vi "UnscentedKalmanFilter_New.vi"(5 "States":i32, 6 "dt_Seconds":dbl=0.02, 7 "Outputs":i32, 8 "UNSCENTED_KALMAN_NEW_FUNC_GROUP":T1, 10 "MeasurementStdDevs":T3, 11 "StateStdDevs":T3) -> (0 "Error":bool, 3 "UnscentedKalmanFiilter":T4)   [LabVIEW 2019, in "Trajectory_Library.lvlib"]
doc: "Creates a new LINEAR SYSTEM data cluster with the specified values. \n\n\nInputs: \n - XXX -- XXX.\n\nOutputs:\n - XXX -- XXX."
uses:
  Trajectory_Library.lvlib
  UNSCENTED_KALMAN_FILTER.ctl
  <vilib>/Analysis/Matrix/Datatypes/RealMatrix.ctl
  MERWE_SCALED_SIGMA_PTS.ctl
  BiFunction_FUNC_TYPE.ctl
  UNSCENTED_KALMAN_NEW_FUNC_GROUP.ctl
  MatrixHelper_CoerceSize.vi
  <vilib>/Analysis/Matrix/NI_Matrix.lvlib
panel:
  # "<States,1>"
  # "<Outputs,1>"
  # "State Estimate <Statess,1>"
  # "<States, States>"
  # "<States, ?>"
  # "<Statess,  States>"
  # "<Outputs, Outputs>"
  # "<?, 1>"
  # "<?, 1>"
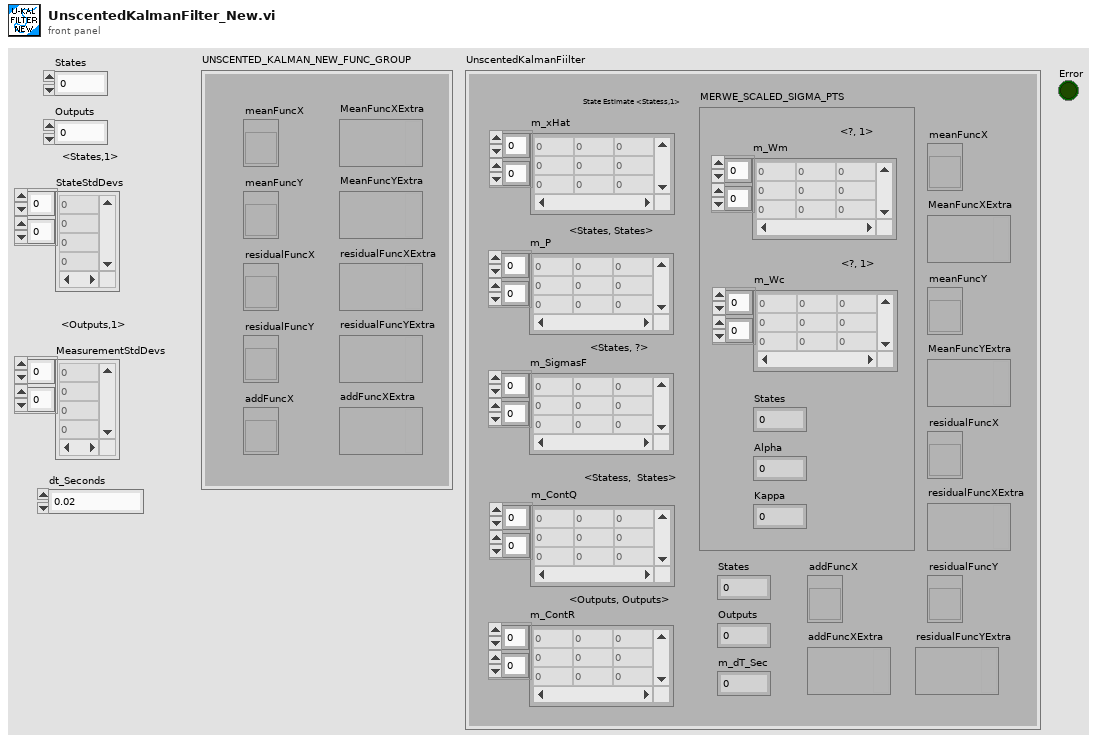
[diagram p1: front panel]
types:
  T1 = typedef "Trajectory_Library.lvlib/UNSCENTED_KALMAN_NEW_FUNC_GROUP.ctl" = cluster{"meanFuncX":T2, "meanFuncY":T2, "residualFuncX":T2, "residualFuncY":T2, "addFuncX":T2, "MeanFuncXExtra":variant, "MeanFuncYExtra":variant, "residualFuncXExtra":variant, "residualFuncYExtra":variant, "addFuncXExtra":variant}
  T2 = typedef "Trajectory_Library.lvlib/BiFunction_FUNC_TYPE.ctl" = refnum<vi>
  T3 = typedef "NI_Matrix.lvlib/RealMatrix.ctl" = dbl[][]
  T4 = typedef "Trajectory_Library.lvlib/UNSCENTED_KALMAN_FILTER.ctl" = cluster{"m_P":T3, "m_xHat":T3, "States":i32, "Outputs":i32, "m_ContR":T3, "m_ContQ":T3, "m_SigmasF":T3, "m_dT_Sec":dbl, "MERWE_SCALED_SIGMA_PTS":T5, "meanFuncX":T2, "meanFuncY":T2, "residualFuncX":T2, "residualFuncY":T2, "addFuncX":T2, "addFuncXExtra":variant, "residualFuncYExtra":variant, "residualFuncXExtra":variant, "MeanFuncYExtra":variant, "MeanFuncXExtra":variant}
  T5 = typedef "Trajectory_Library.lvlib/MERWE_SCALED_SIGMA_PTS.ctl" = cluster{"m_Wm":T3, "States":i32, "Alpha":dbl, "m_Wc":T3, "Kappa":i32}
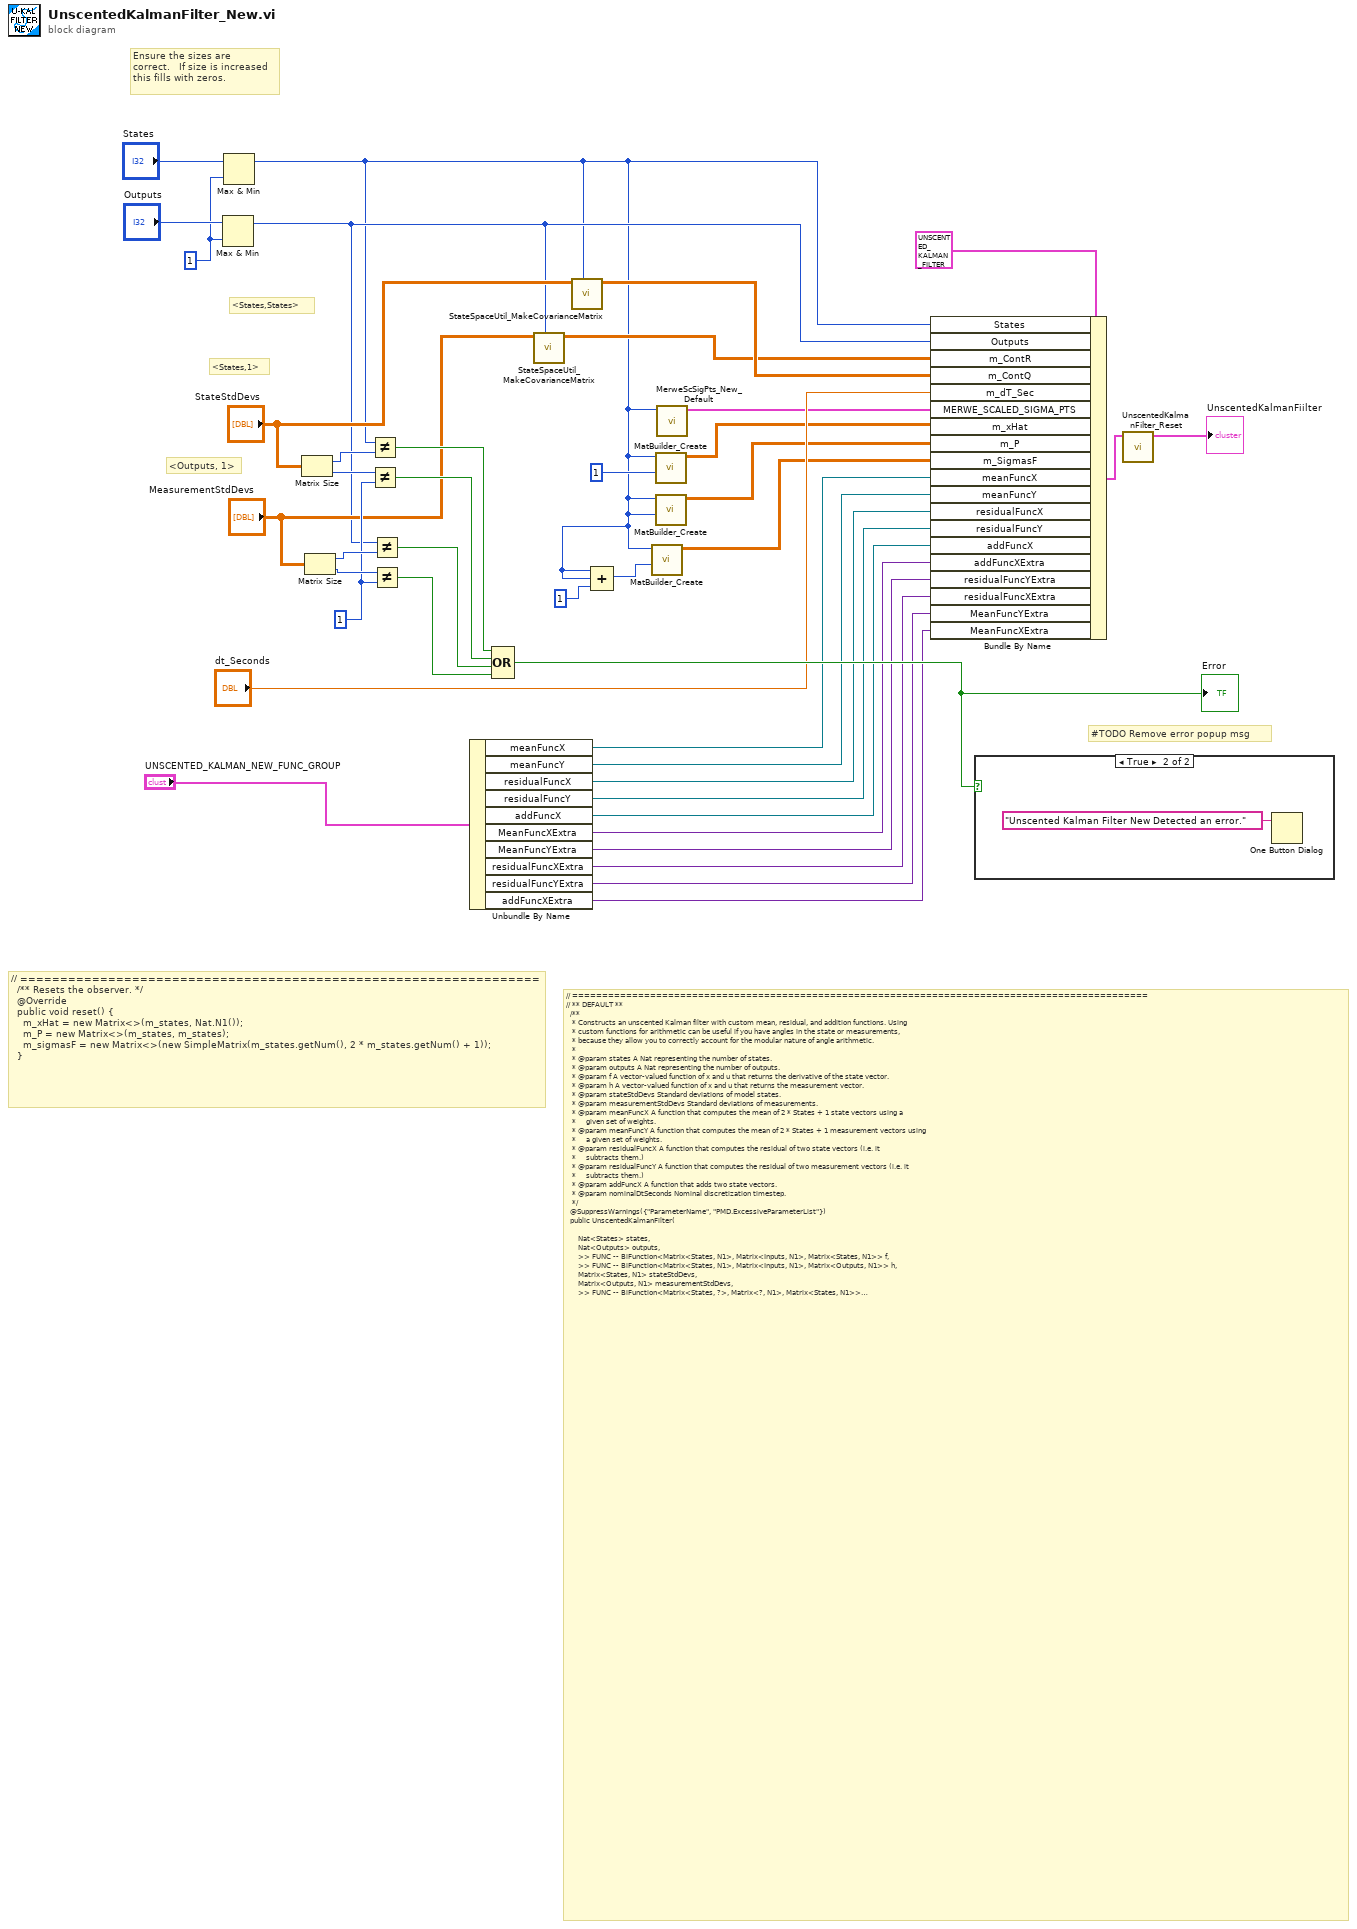
[diagram p0: block diagram]
diagram:
  w30 = 1 ("y")
  w39 = 1 ("y")
  # "// =================================================================\n  /** Resets the observer. */\n  @Override\n  public void reset() {\n    m_xHat = new Matrix<>(m_states, Nat.N1());\n    m_P = new Matrix<>(m_states, m_states);\n    m_sigmasF = new Matrix<>(new SimpleMatrix(m_states.getNum(), 2 * m_states.getNum() + 1));\n  }"
  # "// ================================================================================================\n// ** DEFAULT **\n  /**\n   * Constructs an unscented Kalman filter with custom mean, residual, and addition functions. Using\n   * custom functions for arithmetic can be useful if you have angles in the state or measurements,\n   * because they allow you to correctly account for the modular nature of angle arithmetic.\n   *\n   * @param states A Nat representing the number of states.\n   * @param outputs A Nat representing the number of outputs.\n   * @param f A vector-valued function of x and u that returns the derivative of the state vector.\n   * @param h A vector-valued function of x and u that returns the measurement vector.\n   * @param stateStdDevs Standard deviations of model states.\n   * @param measurementStdDevs Standard deviations of measurements.\n   * @param meanFuncX A function that computes the mean of 2 * States + 1 state vectors using a\n   *     given set of weights.\n   * @param meanFuncY A function that computes the mean of 2 * States + 1 measurement vectors using\n   *     a given set of weights.\n   * @param residualFuncX A function that computes the residual of two state vectors (i.e. it\n   *     subtracts them.)\n   * @param residualFuncY A function that computes the residual of two measurement vectors (i.e. it\n   *     subtracts them.)\n   * @param addFuncX A function that adds two state vectors.\n   * @param nominalDtSeconds Nominal discretization timestep.\n   */\n  @SuppressWarnings({\"ParameterName\", \"PMD.ExcessiveParameterList\"})\n  public UnscentedKalmanFilter(\n\n      Nat<States> states,\n      Nat<Outputs> outputs,\n      >> FUNC -- BiFunction<Matrix<States, N1>, Matrix<Inputs, N1>, Matrix<States, N1>> f,\n      >> FUNC -- BiFunction<Matrix<States, N1>, Matrix<Inputs, N1>, Matrix<Outputs, N1>> h,\n      Matrix<States, N1> stateStdDevs,\n      Matrix<Outputs, N1> measurementStdDevs,\n      >> FUNC -- BiFunction<Matrix<States, ?>, Matrix<?, N1>, Matrix<States, N1>> meanFuncX,\n      >> FUNC -- BiFunction<Matrix<Outputs, ?>, Matrix<?, N1>, Matrix<Outputs, N1>> meanFuncY,\n      >> FUNC -- BiFunction<Matrix<States, N1>, Matrix<States, N1>, Matrix<States, N1>> residualFuncX,\n      >> FUNC -- BiFunction<Matrix<Outputs, N1>, Matrix<Outputs, N1>, Matrix<Outputs, N1>> residualFuncY,\n      >> FUNC -- BiFunction<Matrix<States, N1>, Matrix<States, N1>, Matrix<States, N1>> addFuncX,\n      double nominalDtSeconds) {\n\n    this.m_states = states;\n    this.m_outputs = outputs;\n\n    m_f = f;\n    m_h = h;\n\n    m_meanFuncX = meanFuncX;\n    m_meanFuncY = meanFuncY;\n    m_residualFuncX = residualFuncX;\n    m_residualFuncY = residualFuncY;\n    m_addFuncX = addFuncX;\n\n    m_dtSeconds = nominalDtSeconds;\n\n    m_contQ = StateSpaceUtil.makeCovarianceMatrix(states, stateStdDevs);\n    m_contR = StateSpaceUtil.makeCovarianceMatrix(outputs, measurementStdDevs);\n\n    m_pts = new MerweScaledSigmaPoints<>(states);\n\n    reset();\n  }"
  # "#TODO Remove error popup msg"
  # "<Outputs, 1>"
  # "<States,1>"
  # "<States,States>"
  # "Ensure the sizes are\ncorrect.   If size is increased \nthis fills with zeros."
  n1 = Max & Min(x="Outputs", y=w39) -> (max(x,y)=w23:i32)  [unwired: 1 out]
  n2 = Max & Min(x="States", y=w39) -> (max(x,y)=w14:i32)  [unwired: 1 out]
  n3 = Matrix Size(0:"StateStdDevs") -> (1:w38:i32, 2:w35:i32)
  n4 = Matrix Size(0:"MeasurementStdDevs") -> (1:w36:i32, 2:w37:i32)
  n5 = Not Equal?(x=w14, y=w38) -> (x != y?=w31:bool)
  n6 = Not Equal?(x=w35, y=w30) -> (x != y?=w32:bool)
  n7 = Not Equal?(x=w23, y=w36) -> (x != y?=w33:bool)
  n8 = Not Equal?(x=w37, y=w30) -> (x != y?=w34:bool)
  n9 = Unbundle By Name("UNSCENTED_KALMAN_NEW_FUNC_GROUP") -> ("meanFuncX"=w10:T2, "meanFuncY"=w9:T2, "residualFuncX"=w8:T2, "residualFuncY"=w7:T2, "addFuncX"=w6:T2, "MeanFuncXExtra"=w5:variant, "MeanFuncYExtra"=w4:variant, "residualFuncXExtra"=w3:variant, "residualFuncYExtra"=w2:variant, "addFuncXExtra"=w1:variant)
  n10 = Compound Arithmetic op=OR(w31, w32, w33, w34) -> (w29:bool)
  "Error" <- w29
  n11 = call "StateSpaceUtil_MakeCovarianceMatrix.vi"("States"=w23, "StdDevs"="MeasurementStdDevs") -> ("Covariance Matrix"=w22:T3)  [unwired: 9 in]
  n12 = call "StateSpaceUtil_MakeCovarianceMatrix.vi"("States"=w14, "StdDevs"="StateStdDevs") -> ("Covariance Matrix"=w25:T3)  [unwired: 9 in]
  n13 = Compound Arithmetic op=ADD(w14, w14, 1 ("value")) -> (w13:i32)
  n14 = call "MatBuilder_Create.vi"("Columns"=w13, "Rows"=w14) -> ("output matrix"=w12:T3)  [unwired: 9 in]
  n15 = call "MatBuilder_Create.vi"("Columns"=1, "Rows"=w14) -> ("output matrix"=w17:T3)  [unwired: 9 in]
  n16 = call "MatBuilder_Create.vi"("Columns"=w14, "Rows"=w14) -> ("output matrix"=w16:T3)  [unwired: 9 in]
  n17 = call "MerweScSigPts_New_Default.vi"("States"=w14) -> ("MerweScaledSigmaPts"=w21:T5)  [unwired: 10 in]
  n18 = Bundle By Name(cluster=T4 {"m_P"=[], "m_xHat"=[], "States"=0, "Outputs"=0, "m_ContR"=[], "m_ContQ"=[], "m_SigmasF"=[], "m_dT_Sec"=0.0, "MERWE_SCALED_SIGMA_PTS"={"m_Wm"=[], "States"=0, "Alpha"=0.0, "m_Wc"=[], "Kappa"=0}, "meanFuncX"=refnum, "meanFuncY"=refnum, "residualFuncX"=refnum, "residualFuncY"=refnum, "addFuncX"=refnum, "addFuncXExtra"=variant, "residualFuncYExtra"=variant, "residualFuncXExtra"=variant, "MeanFuncYExtra"=variant, "MeanFuncXExtra"=variant} ("UNSCENTED_KALMAN_FILTER"), "States"=w14, "Outputs"=w23, "m_ContR"=w22, "m_ContQ"=w25, "m_dT_Sec"="dt_Seconds", "MERWE_SCALED_SIGMA_PTS"=w21, "m_xHat"=w17, "m_P"=w16, "m_SigmasF"=w12, "meanFuncX"=w10, "meanFuncY"=w9, "residualFuncX"=w8, "residualFuncY"=w7, "addFuncX"=w6, "addFuncXExtra"=w5, "residualFuncYExtra"=w4, "residualFuncXExtra"=w3, "MeanFuncYExtra"=w2, "MeanFuncXExtra"=w1) -> (w20:T4)
  n19 = case shown="True" w29 {
    frame False {
    }
    frame True {
      n20 = One Button Dialog(message="Unscented Kalman Filter New Detected an error.") -> ()  [unwired: 1 in, 1 out]
    }
  }
  n21 = call "UnscentedKalmanFilter_Reset.vi"("in UnscentedKalmanFiilter"=w20) -> ("out UnscentedKalmanFiilter"=→"UnscentedKalmanFiilter":T4)  [unwired: 10 in]
